vi "Count True.vi"(7 "Booleans":bool[](array[boolean])) -> (8 "Count":u16)   [LabVIEW 2026]
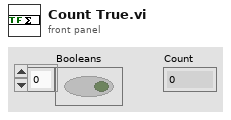
[diagram p1: front panel]
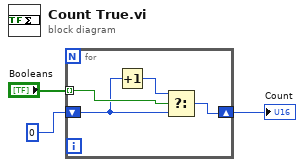
[diagram p0: block diagram]
diagram:
  n1 = for {
    tunnel: "Booleans" -> [w7] mode=indexing
    shift-right: [w4] -> w3
    shift-left: i16 0 -> [w6]
    n2 = Increment(x=w6) -> (x+1=w5:i16)
    n3 = Select(t=w5, s=w7, f=w6) -> (s? t:f=w4:i16)
  }
  "Count" <- w3
